vi "Prevention Table.vi"() -> ()   [LabVIEW 2019]
uses:
  LLB/Commonly VI/Main Glb.vi
  LLB/Commonly VI.lvlib
panel:
  out "ArrivePercentage100":bool[](array[boolean])
  out "Receive PLC Data":i32
  in  "Tab Control":enum32{"Page 1", "Page 2", "Page 3", "Page 4"}(tab)
  out "Array 5":T1[](array[typedef])=[80, 82, 84, 86, 88, 10, 12, 14, 16, 18, 20, 22, 24, 26, 28, 30, 32, 34, 36, 38, 40, 42, 44, 46, 48, 50, 52, 54, 56, 58, 60, 62, 64, 66, 68, 70, 72, 74, 76, 78, 80, 82, 84, 86, 88] items=["0_S1檢平確認氣缸_0", "1_S1檢平確認氣缸_1", "2_S1電路板檢平On次數_0", "3_S1電路板檢平On次數_1", "4_S1 電池檢平On次數_0", "5_S1 電池檢平On次數_1", "6_S1 盒蓋檢平On次數_0", "7_S1 盒蓋檢平On次數_1", "8_S2電流量測探針使用次數_0", "9_S2電流量測探針使用次數_1", "10_S2-電流量測氣缸_0", "11_S2-電流量測氣缸_1", "12_S3程式燒入 探針使用次數_0", "13_S3程式燒入 探針使用次數_1", "14_S3-程式燒入氣缸_0", "15_S3-程式燒入氣缸_1", "16_S4電壓量測探針使用次數_0", "17_S4電壓量測探針使用次數_1", "18_S4電源3V探針使用次數_0", "19_S4電源3V探針使用次數_1", "20_S4-隔離箱上蓋氣缸_0", "21_S4-隔離箱上蓋氣缸_1", "22_S4-隔離箱下蓋氣缸_0", "23_S4-隔離箱下蓋氣缸_1", "24_S4-電池電壓量測固定氣缸_0", "25_S4-電池電壓量測固定氣缸_1", "26_S4-電池電壓量測氣缸_0", "27_S4-電池電壓量測氣缸_1", "28_S4-電路板檢測氣缸_0", "29_S4-電路板檢測氣缸_1", "30_S5-電路板取料升降氣缸_0", "31_S5-電路板取料升降氣缸_1", "32_S5-電路板取料橫移氣缸_0", "33_S5-電路板取料橫移氣缸_1", "34_S5-吸真空_0", "35_S5-吸真空_1", "36_S5-破真空_0", "37_S5-破真空_1", "38_S7-焊接料件固定氣缸_0", "39_S7-焊接料件固定氣缸_1", "40_S7-焊接機清錫馬達_0", "41_S7-焊接機清錫馬達_1", "42_S10-料件翻轉區升降氣缸_0", "43_S10-料件翻轉區升降氣缸_1", "44_S10-料件翻轉區伸出氣缸_0", "45_S10-料件翻轉區伸出氣缸_1", "46_S10-料件翻轉區旋轉氣缸_0", "47_S10-料件翻轉區旋轉氣缸_1", "48_S10-料件翻轉區夾取氣缸_0", "49_S10-料件翻轉區夾取氣缸_1", "50_S10-料件橫移氣缸_0", "51_S10-料件橫移氣缸_1", "52_S10-料件吸取升降氣缸_0", "53_S10-料件吸取升降氣缸_1", "54_S10-料件放料升降氣缸_0", "55_S10-料件放料升降氣缸_1", "56_S10-吸真空_0", "57_S10-吸真空_1", "58_S10-破真空_0", "59_S10-破真空_1", "60_S11-雷射測高檢知氣缸_0", "61_S11-雷射測高檢知氣缸_1", "62_S12-熱熔升降氣缸_0", "63_S12-熱熔升降氣缸_1", "64_S12-預熱升降氣缸_0", "65_S12-預熱升降氣缸_1", "66_S12-離子槍風速調控_0", "67_S12-離子槍風速調控_1", "68_S13-吸真空_0", "69_S13-吸真空_1", "70_S13-破真空_0", "71_S13-破真空_1", "72_S13-NG蓋取料夾爪_0", "73_S13-NG蓋取料夾爪_1", "74_S13-NG蓋取料升降_0", "75_S13-NG蓋取料升降_1", "76_S13-NG電池取料升降_0", "77_S13-NG電池取料升降_1", "78_S13-NG電路板取料升降_0", "79_S13-NG電路板取料升降_1", "80_S13-NG橫移氣缸_0", "81_S13-NG橫移氣缸_1", "82_S13-NG橫移氣缸_0", "83_S13-NG橫移氣缸_1", "84_S7-焊接啟動次數_0", "85_S7-焊接啟動次數_1", "86_S12-熱熔次數_0", "87_S12-熱熔次數_1", "88_S11-雷射檢測次數_0", "89_S11-雷射檢測次數_1"]
  out "Array 4":T1[](array[typedef])=[40, 42, 44, 46, 48, 50, 52, 54, 56, 58, 60, 62, 64, 66, 68, 70, 72, 74, 76, 78, 40, 42, 44, 46, 48, 50, 52, 54, 56, 58, 60, 62, 64, 66, 68, 70, 72, 74, 76, 78, 80, 82, 84, 86, 88] items=["0_S1檢平確認氣缸_0", "1_S1檢平確認氣缸_1", "2_S1電路板檢平On次數_0", "3_S1電路板檢平On次數_1", "4_S1 電池檢平On次數_0", "5_S1 電池檢平On次數_1", "6_S1 盒蓋檢平On次數_0", "7_S1 盒蓋檢平On次數_1", "8_S2電流量測探針使用次數_0", "9_S2電流量測探針使用次數_1", "10_S2-電流量測氣缸_0", "11_S2-電流量測氣缸_1", "12_S3程式燒入 探針使用次數_0", "13_S3程式燒入 探針使用次數_1", "14_S3-程式燒入氣缸_0", "15_S3-程式燒入氣缸_1", "16_S4電壓量測探針使用次數_0", "17_S4電壓量測探針使用次數_1", "18_S4電源3V探針使用次數_0", "19_S4電源3V探針使用次數_1", "20_S4-隔離箱上蓋氣缸_0", "21_S4-隔離箱上蓋氣缸_1", "22_S4-隔離箱下蓋氣缸_0", "23_S4-隔離箱下蓋氣缸_1", "24_S4-電池電壓量測固定氣缸_0", "25_S4-電池電壓量測固定氣缸_1", "26_S4-電池電壓量測氣缸_0", "27_S4-電池電壓量測氣缸_1", "28_S4-電路板檢測氣缸_0", "29_S4-電路板檢測氣缸_1", "30_S5-電路板取料升降氣缸_0", "31_S5-電路板取料升降氣缸_1", "32_S5-電路板取料橫移氣缸_0", "33_S5-電路板取料橫移氣缸_1", "34_S5-吸真空_0", "35_S5-吸真空_1", "36_S5-破真空_0", "37_S5-破真空_1", "38_S7-焊接料件固定氣缸_0", "39_S7-焊接料件固定氣缸_1", "40_S7-焊接機清錫馬達_0", "41_S7-焊接機清錫馬達_1", "42_S10-料件翻轉區升降氣缸_0", "43_S10-料件翻轉區升降氣缸_1", "44_S10-料件翻轉區伸出氣缸_0", "45_S10-料件翻轉區伸出氣缸_1", "46_S10-料件翻轉區旋轉氣缸_0", "47_S10-料件翻轉區旋轉氣缸_1", "48_S10-料件翻轉區夾取氣缸_0", "49_S10-料件翻轉區夾取氣缸_1", "50_S10-料件橫移氣缸_0", "51_S10-料件橫移氣缸_1", "52_S10-料件吸取升降氣缸_0", "53_S10-料件吸取升降氣缸_1", "54_S10-料件放料升降氣缸_0", "55_S10-料件放料升降氣缸_1", "56_S10-吸真空_0", "57_S10-吸真空_1", "58_S10-破真空_0", "59_S10-破真空_1", "60_S11-雷射測高檢知氣缸_0", "61_S11-雷射測高檢知氣缸_1", "62_S12-熱熔升降氣缸_0", "63_S12-熱熔升降氣缸_1", "64_S12-預熱升降氣缸_0", "65_S12-預熱升降氣缸_1", "66_S12-離子槍風速調控_0", "67_S12-離子槍風速調控_1", "68_S13-吸真空_0", "69_S13-吸真空_1", "70_S13-破真空_0", "71_S13-破真空_1", "72_S13-NG蓋取料夾爪_0", "73_S13-NG蓋取料夾爪_1", "74_S13-NG蓋取料升降_0", "75_S13-NG蓋取料升降_1", "76_S13-NG電池取料升降_0", "77_S13-NG電池取料升降_1", "78_S13-NG電路板取料升降_0", "79_S13-NG電路板取料升降_1", "80_S13-NG橫移氣缸_0", "81_S13-NG橫移氣缸_1", "82_S13-NG橫移氣缸_0", "83_S13-NG橫移氣缸_1", "84_S7-焊接啟動次數_0", "85_S7-焊接啟動次數_1", "86_S12-熱熔次數_0", "87_S12-熱熔次數_1", "88_S11-雷射檢測次數_0", "89_S11-雷射檢測次數_1"]
  out "Array 3":T1[](array[typedef])=[0, 2, 4, 6, 8, 10, 12, 14, 16, 18, 20, 22, 24, 26, 28, 30, 32, 34, 36, 38, 40, 42, 44, 46, 48, 50, 52, 54, 56, 58, 60, 62, 64, 66, 68, 70, 72, 74, 76, 78, 80, 82, 84, 86, 88] items=["0_S1檢平確認氣缸_0", "1_S1檢平確認氣缸_1", "2_S1電路板檢平On次數_0", "3_S1電路板檢平On次數_1", "4_S1 電池檢平On次數_0", "5_S1 電池檢平On次數_1", "6_S1 盒蓋檢平On次數_0", "7_S1 盒蓋檢平On次數_1", "8_S2電流量測探針使用次數_0", "9_S2電流量測探針使用次數_1", "10_S2-電流量測氣缸_0", "11_S2-電流量測氣缸_1", "12_S3程式燒入 探針使用次數_0", "13_S3程式燒入 探針使用次數_1", "14_S3-程式燒入氣缸_0", "15_S3-程式燒入氣缸_1", "16_S4電壓量測探針使用次數_0", "17_S4電壓量測探針使用次數_1", "18_S4電源3V探針使用次數_0", "19_S4電源3V探針使用次數_1", "20_S4-隔離箱上蓋氣缸_0", "21_S4-隔離箱上蓋氣缸_1", "22_S4-隔離箱下蓋氣缸_0", "23_S4-隔離箱下蓋氣缸_1", "24_S4-電池電壓量測固定氣缸_0", "25_S4-電池電壓量測固定氣缸_1", "26_S4-電池電壓量測氣缸_0", "27_S4-電池電壓量測氣缸_1", "28_S4-電路板檢測氣缸_0", "29_S4-電路板檢測氣缸_1", "30_S5-電路板取料升降氣缸_0", "31_S5-電路板取料升降氣缸_1", "32_S5-電路板取料橫移氣缸_0", "33_S5-電路板取料橫移氣缸_1", "34_S5-吸真空_0", "35_S5-吸真空_1", "36_S5-破真空_0", "37_S5-破真空_1", "38_S7-焊接料件固定氣缸_0", "39_S7-焊接料件固定氣缸_1", "40_S7-焊接機清錫馬達_0", "41_S7-焊接機清錫馬達_1", "42_S10-料件翻轉區升降氣缸_0", "43_S10-料件翻轉區升降氣缸_1", "44_S10-料件翻轉區伸出氣缸_0", "45_S10-料件翻轉區伸出氣缸_1", "46_S10-料件翻轉區旋轉氣缸_0", "47_S10-料件翻轉區旋轉氣缸_1", "48_S10-料件翻轉區夾取氣缸_0", "49_S10-料件翻轉區夾取氣缸_1", "50_S10-料件橫移氣缸_0", "51_S10-料件橫移氣缸_1", "52_S10-料件吸取升降氣缸_0", "53_S10-料件吸取升降氣缸_1", "54_S10-料件放料升降氣缸_0", "55_S10-料件放料升降氣缸_1", "56_S10-吸真空_0", "57_S10-吸真空_1", "58_S10-破真空_0", "59_S10-破真空_1", "60_S11-雷射測高檢知氣缸_0", "61_S11-雷射測高檢知氣缸_1", "62_S12-熱熔升降氣缸_0", "63_S12-熱熔升降氣缸_1", "64_S12-預熱升降氣缸_0", "65_S12-預熱升降氣缸_1", "66_S12-離子槍風速調控_0", "67_S12-離子槍風速調控_1", "68_S13-吸真空_0", "69_S13-吸真空_1", "70_S13-破真空_0", "71_S13-破真空_1", "72_S13-NG蓋取料夾爪_0", "73_S13-NG蓋取料夾爪_1", "74_S13-NG蓋取料升降_0", "75_S13-NG蓋取料升降_1", "76_S13-NG電池取料升降_0", "77_S13-NG電池取料升降_1", "78_S13-NG電路板取料升降_0", "79_S13-NG電路板取料升降_1", "80_S13-NG橫移氣缸_0", "81_S13-NG橫移氣缸_1", "82_S13-NG橫移氣缸_0", "83_S13-NG橫移氣缸_1", "84_S7-焊接啟動次數_0", "85_S7-焊接啟動次數_1", "86_S12-熱熔次數_0", "87_S12-熱熔次數_1", "88_S11-雷射檢測次數_0", "89_S11-雷射檢測次數_1"]
  out "1_20":i32[](array[numeric]) caption="1~20"
  out "21_40":i32[](array[numeric]) caption="21~40"
  out "41_45":i32[](array[numeric]) caption="41~45"
  out "Array 7":i32[](array[numeric])=[1, 2, 3, 4, 5, 6, 7, 8, 9, 10, 11, 12, 13, 14, 15, 16, 17, 18, 19, 20]
  out "Percentage 80":bool[](array[boolean])
  out "Percentage 81":bool[](array[boolean])
  out "Percentage 82":bool[](array[boolean])
  # "次數達"
  # "次數達"
  # "次數達"
  # "80%"
  # "80%"
  # "80%"
  # "項次"
  # "預防保養次數顯示"
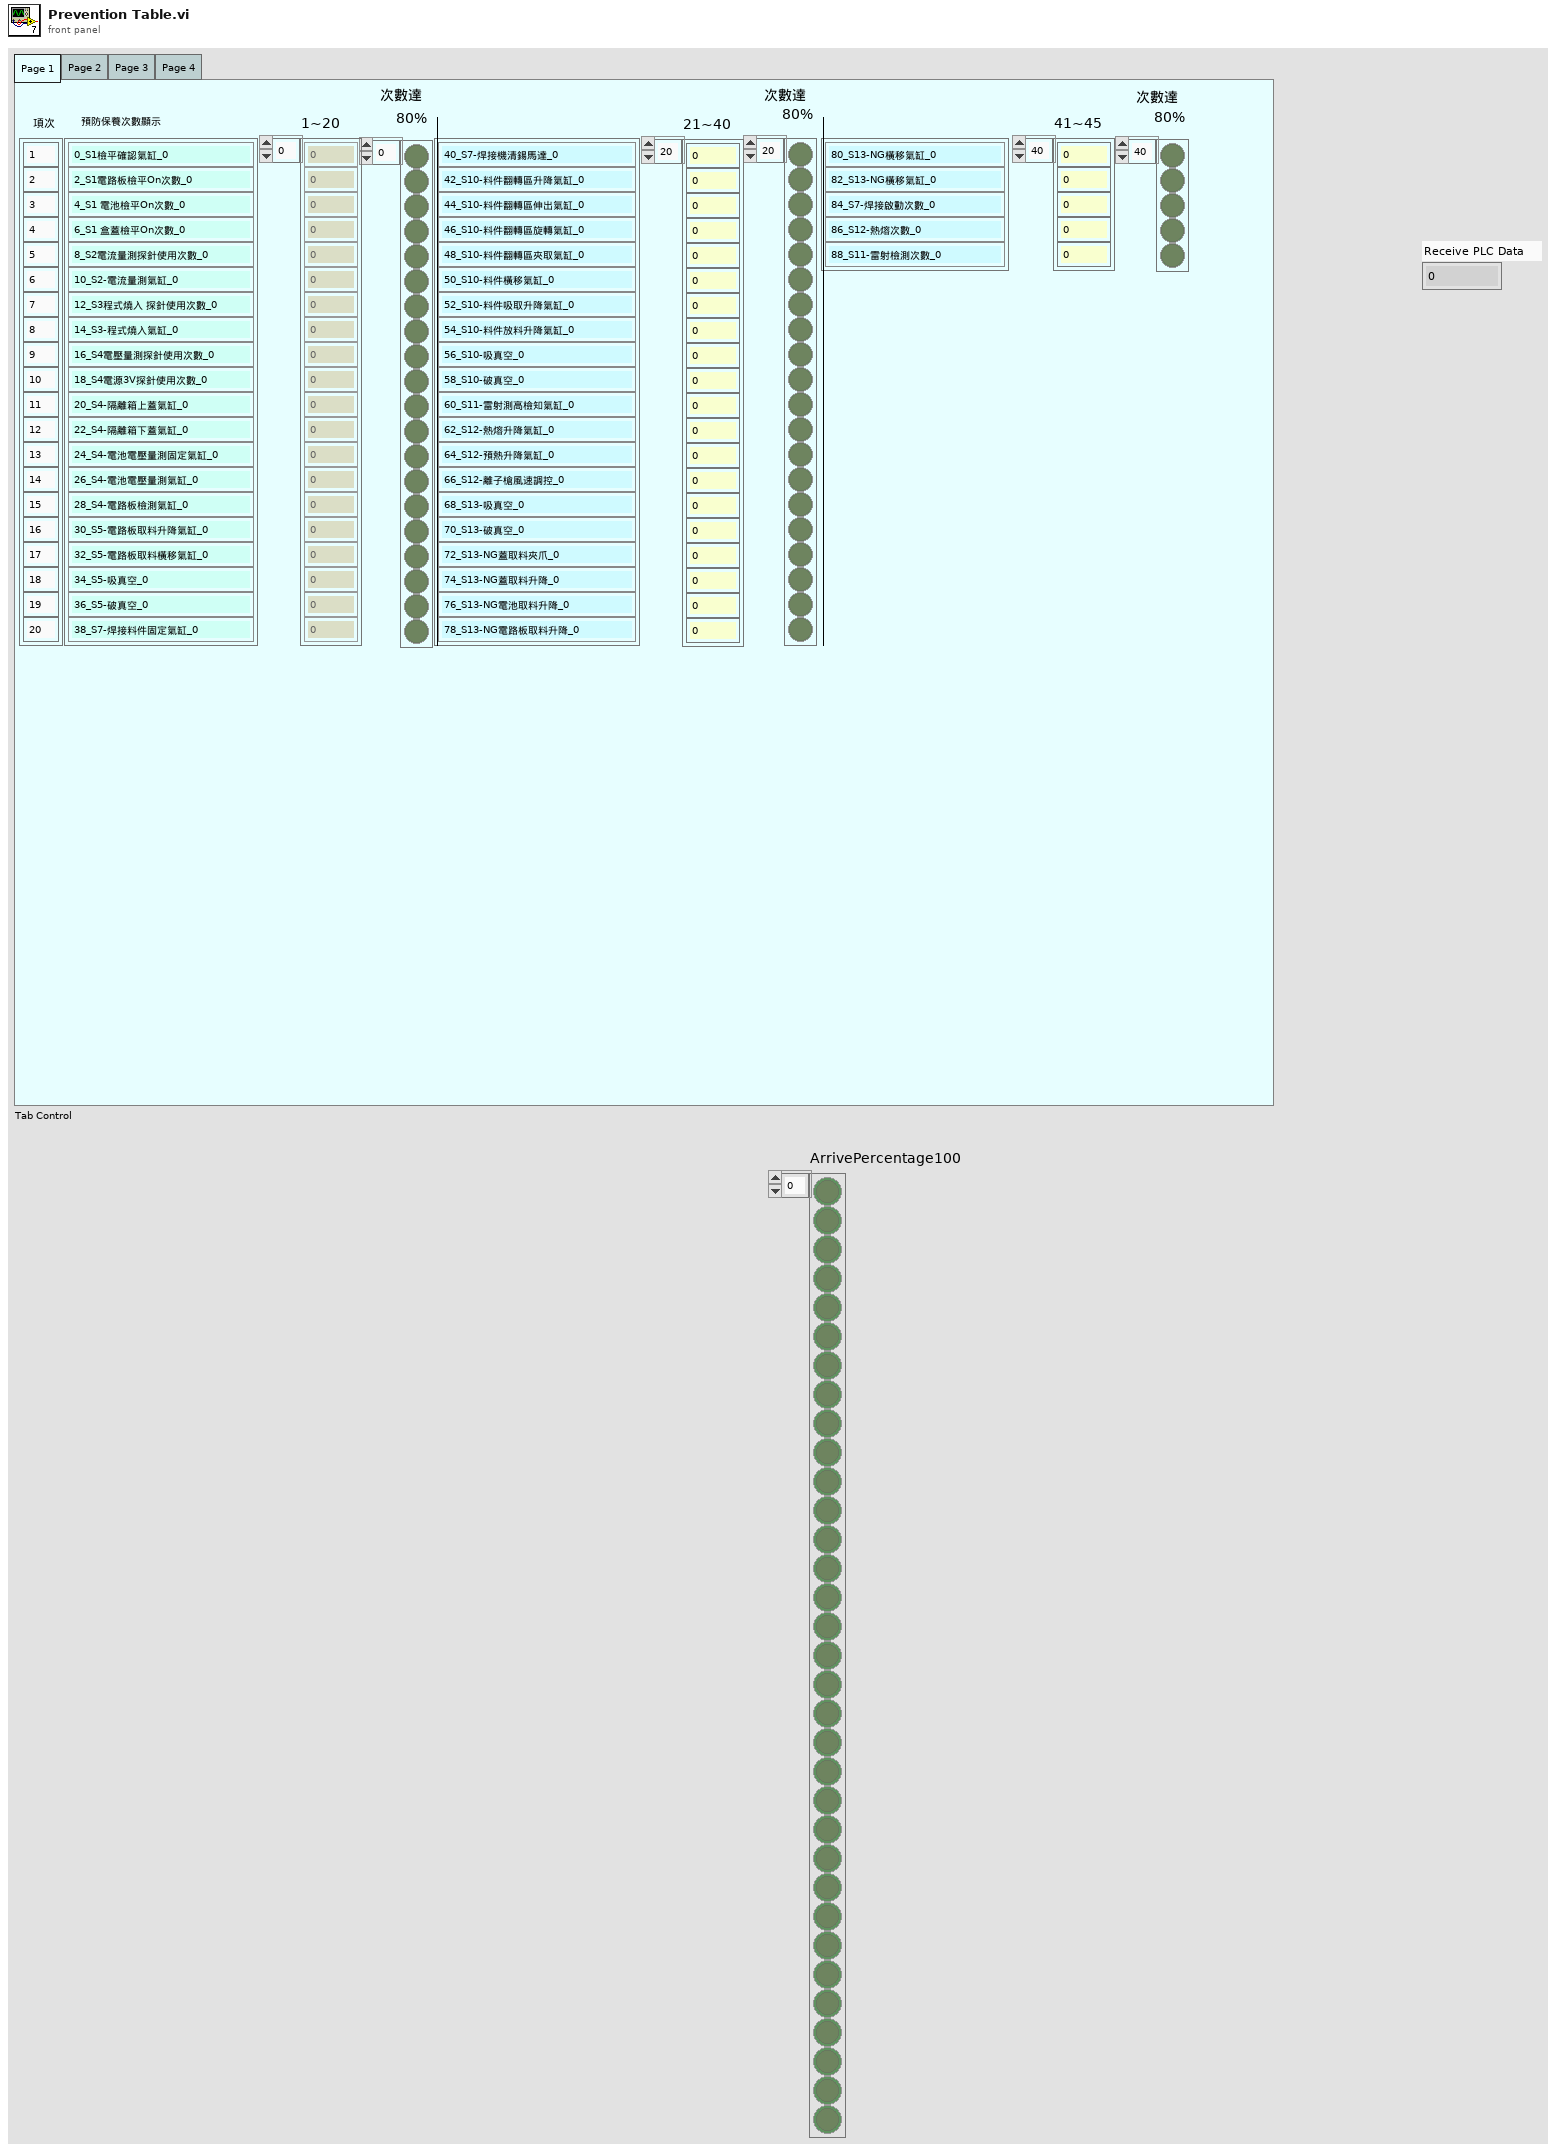
[diagram p1: front panel]
types:
  T1 = typedef "預防保養02.ctl" = u16
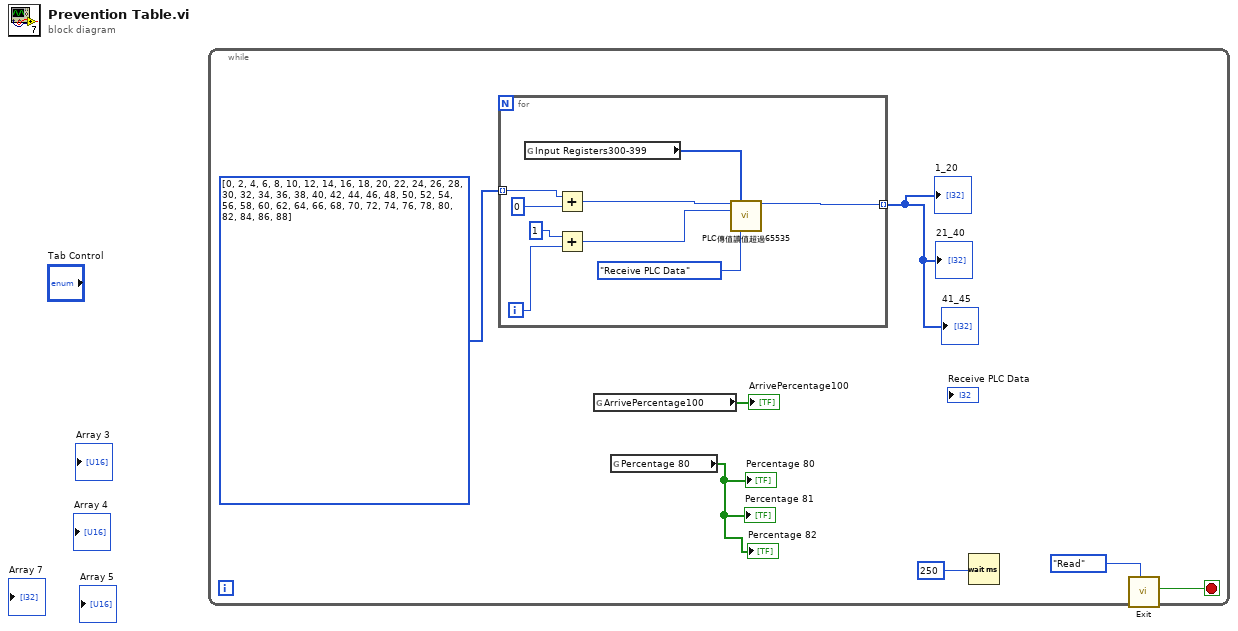
[diagram p0: block diagram]
diagram:
  n1 = while {
    stop <- w6 stop-if-true
    w4 = T1[] [0, 2, 4, 6, 8, 10, 12, 14, 16, 18, 20, 22, 24, 26, 28, 30, 32, 34, 36, 38, 40, 42, 44, 46, 48, 50, 52, 54, 56, 58, 60, 62, 64, 66, 68, 70, 72, 74, 76, 78, 80, 82, 84, 86, 88] items=["0_S1檢平確認氣缸_0", "1_S1檢平確認氣缸_1", "2_S1電路板檢平On次數_0", "3_S1電路板檢平On次數_1", "4_S1 電池檢平On次數_0", "5_S1 電池檢平On次數_1", "6_S1 盒蓋檢平On次數_0", "7_S1 盒蓋檢平On次數_1", "8_S2電流量測探針使用次數_0", "9_S2電流量測探針使用次數_1", "10_S2-電流量測氣缸_0", "11_S2-電流量測氣缸_1", "12_S3程式燒入 探針使用次數_0", "13_S3程式燒入 探針使用次數_1", "14_S3-程式燒入氣缸_0", "15_S3-程式燒入氣缸_1", "16_S4電壓量測探針使用次數_0", "17_S4電壓量測探針使用次數_1", "18_S4電源3V探針使用次數_0", "19_S4電源3V探針使用次數_1", "20_S4-隔離箱上蓋氣缸_0", "21_S4-隔離箱上蓋氣缸_1", "22_S4-隔離箱下蓋氣缸_0", "23_S4-隔離箱下蓋氣缸_1", "24_S4-電池電壓量測固定氣缸_0", "25_S4-電池電壓量測固定氣缸_1", "26_S4-電池電壓量測氣缸_0", "27_S4-電池電壓量測氣缸_1", "28_S4-電路板檢測氣缸_0", "29_S4-電路板檢測氣缸_1", "30_S5-電路板取料升降氣缸_0", "31_S5-電路板取料升降氣缸_1", "32_S5-電路板取料橫移氣缸_0", "33_S5-電路板取料橫移氣缸_1", "34_S5-吸真空_0", "35_S5-吸真空_1", "36_S5-破真空_0", "37_S5-破真空_1", "38_S7-焊接料件固定氣缸_0", "39_S7-焊接料件固定氣缸_1", "40_S7-焊接機清錫馬達_0", "41_S7-焊接機清錫馬達_1", "42_S10-料件翻轉區升降氣缸_0", "43_S10-料件翻轉區升降氣缸_1", "44_S10-料件翻轉區伸出氣缸_0", "45_S10-料件翻轉區伸出氣缸_1", "46_S10-料件翻轉區旋轉氣缸_0", "47_S10-料件翻轉區旋轉氣缸_1", "48_S10-料件翻轉區夾取氣缸_0", "49_S10-料件翻轉區夾取氣缸_1", "50_S10-料件橫移氣缸_0", "51_S10-料件橫移氣缸_1", "52_S10-料件吸取升降氣缸_0", "53_S10-料件吸取升降氣缸_1", "54_S10-料件放料升降氣缸_0", "55_S10-料件放料升降氣缸_1", "56_S10-吸真空_0", "57_S10-吸真空_1", "58_S10-破真空_0", "59_S10-破真空_1", "60_S11-雷射測高檢知氣缸_0", "61_S11-雷射測高檢知氣缸_1", "62_S12-熱熔升降氣缸_0", "63_S12-熱熔升降氣缸_1", "64_S12-預熱升降氣缸_0", "65_S12-預熱升降氣缸_1", "66_S12-離子槍風速調控_0", "67_S12-離子槍風速調控_1", "68_S13-吸真空_0", "69_S13-吸真空_1", "70_S13-破真空_0", "71_S13-破真空_1", "72_S13-NG蓋取料夾爪_0", "73_S13-NG蓋取料夾爪_1", "74_S13-NG蓋取料升降_0", "75_S13-NG蓋取料升降_1", "76_S13-NG電池取料升降_0", "77_S13-NG電池取料升降_1", "78_S13-NG電路板取料升降_0", "79_S13-NG電路板取料升降_1", "80_S13-NG橫移氣缸_0", "81_S13-NG橫移氣缸_1", "82_S13-NG橫移氣缸_0", "83_S13-NG橫移氣缸_1", "84_S7-焊接啟動次數_0", "85_S7-焊接啟動次數_1", "86_S12-熱熔次數_0", "87_S12-熱熔次數_1", "88_S11-雷射檢測次數_0", "89_S11-雷射檢測次數_1"]
    n2 = for {
      tunnel: [w13] -> w3 mode=indexing
      tunnel: w4 -> [w10] mode=indexing
      i -> [w15]
      n3 = global read "Main Glb.vi" "Input Registers300-399"() -> (w8:u16[])
      n4 = Add(x=w10, y=0) -> (x+y=w9:i32)
      n5 = Add(x=1, y=w15) -> (x+y=w12:i32)
      n6 = call "PLC傳值讀值超過65535.vi"("Read PLC Reg Index0"=w9, "Input Registers"=w8, "Read PLC Reg Index1"=w12, "Enum"=enum16{"Send PLC Data", "Receive PLC Data"}."Receive PLC Data") -> ("Receive PLC Data"=w13:i32)  [unwired: 9 in, 2 out]
    }
    "1_20" <- w3
    "21_40" <- w3
    "41_45" <- w3
    n7 = global read "Main Glb.vi" "ArrivePercentage100"() -> (→"ArrivePercentage100":bool[])
    n8 = global read "Main Glb.vi" "Percentage 80"() -> (→"Percentage 80" →"Percentage 81" →"Percentage 82":bool[])
    n9 = Wait (ms)(milliseconds to wait=250) -> ()  [unwired: 1 out]
    n10 = call "Exit.vi"("Enum"=enum16{"Initial", "Read", "Write"}."Read") -> ("ExitOut"=w6:bool)  [unwired: 10 in]
  }
